vi "DAC Init Results.vi"(8 "error in":errorcluster, 9 "Log Details?":bool, 10 "tdms file":refnum<k34>, 11 "DAC DC Supply in":refnum<class "DAC DC Supply.lvclass">) -> (0 "error out":errorcluster, 2 "tdms file out":refnum<k34>)   [LabVIEW 2019, in "DAC.lvlib" / "DAC DC Supply.lvclass"]
uses:
  DAC DC Supply.lvclass
  DAC.lvclass
  C:/Users/wg/Documents/LV_Projects/test-stand/App/DAC/DAC.lvclass
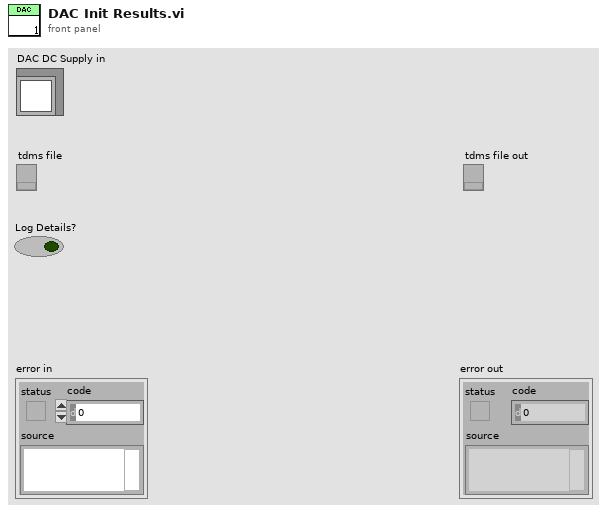
[diagram p1: front panel]
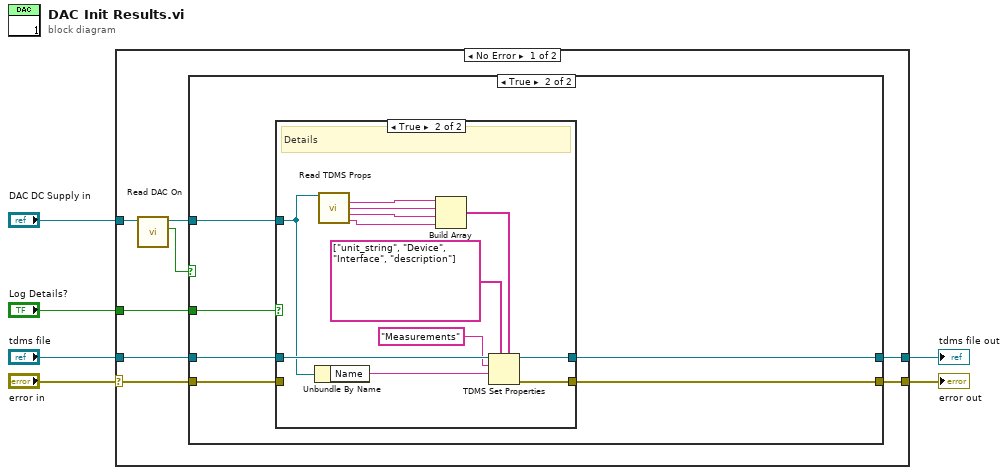
[diagram p0: block diagram]
diagram:
  n1 = case shown="No Error" "error in" {
    selector: "error in" -> [w10 w38]
    tunnel: [w7 w38] -> w1
    tunnel: "DAC DC Supply in" -> [w14 _]
    tunnel: "tdms file" -> [w11 w37]
    tunnel: [w8 w37] -> w2
    tunnel: "Log Details?" -> [w9 _]
    frame No Error {
      n2 = call "Read DAC On.vi"("DAC in"=w14) -> ("DAC On"=w12:bool, "DAC out"=w13:refnum<class "DAC DC Supply.lvclass">)  [unwired: 8 in, 1 out]
      n3 = case shown="True" w12 {
        tunnel: w11 -> [w15 w22]
        tunnel: [w15 w19] -> w8
        tunnel: [w16 w18] -> w7
        tunnel: w13 -> [_ w21]
        tunnel: w10 -> [w16 w17]
        tunnel: w9 -> [_ w20]
        frame False {
        }
        frame True {
          n4 = case shown="True" w20 {
            tunnel: w22 -> [w24 w36]
            tunnel: [w24 w34] -> w19
            tunnel: [w23 w33] -> w18
            tunnel: w21 -> [_ w28]
            tunnel: w17 -> [w23 _]
            frame False {
            }
            frame True {
              # "Details"
              n5 = Unbundle By Name(w28) -> ("Name"=w32:string)
              n6 = call "Read TDMS Props.vi"("DAC in"=w28) -> ("Result Unit"=w29:string, "DAC Device"=w27:string, "DAC IO"=w26:string, "DAC Description"=w25:string)  [unwired: 10 in, 1 out]
              n7 = Build Array(w29, w27, w26, w25) -> (w30:string[])
              n8 = TDMS Set Properties(5:w30, 7:string[] ["unit_string", "Device", "Interface", "description"] ("property names"), 9:w32, 10:"Measurements" ("group name in (Untitled)"), 11:w36) -> (0:w33:errorcluster, 3:w34:refnum<k34>)  [unwired: 1 in, 2 out]
            }
          }
        }
      }
    }
    frame Error {
    }
  }
  "error out" <- w1
  "tdms file out" <- w2
